vi "RCDAQ Voltage Sweep.vi"() -> ()   [LabVIEW 2023]
doc: "This example shows how to configure a measurement and take a reading."
uses:
  <vilib>/net/SSH/Client/PuTTY/PuTTY Client.lvclass
  C:/Program Files/National Instruments/LabVIEW 2023/vi.lib/net/SSH/Client/Generic/Generic Client.lvclass
  Keithley 2450.lvlib
  <vilib>/net/SSH/NI_SSH.lvlib
panel:
  in  "DRS4 Tme (s)":dbl
  in  "Sweep Points":T1={"Start "=1.0, "Stop "=0.0, "Number of Points (5)"=5}
  out "Error":string
  out "Linux Output":string
  in  "Linux Command":string
  out "Current Voltage":string
  in  "Compliance Level (0.1)":dbl=0.1
  in  "Source Mode  (0: Voltage)":u16(ring) items=["Voltage", "Current"]
  in  "VISA resource name":refnum<visa-resource-name>
  # "(c) 2006 National Instruments.  ALL RIGHTS RESERVED."
  # "(c) 2021 National Instruments.  ALL RIGHTS RESERVED."
  # "Source Settings"
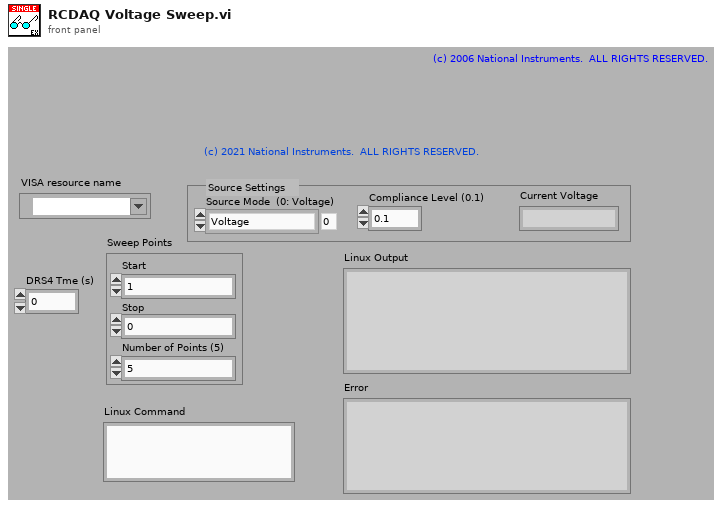
[diagram p1: front panel]
types:
  T1 = cluster{"Start ":dbl, "Stop ":dbl, "Number of Points (5)":u32}
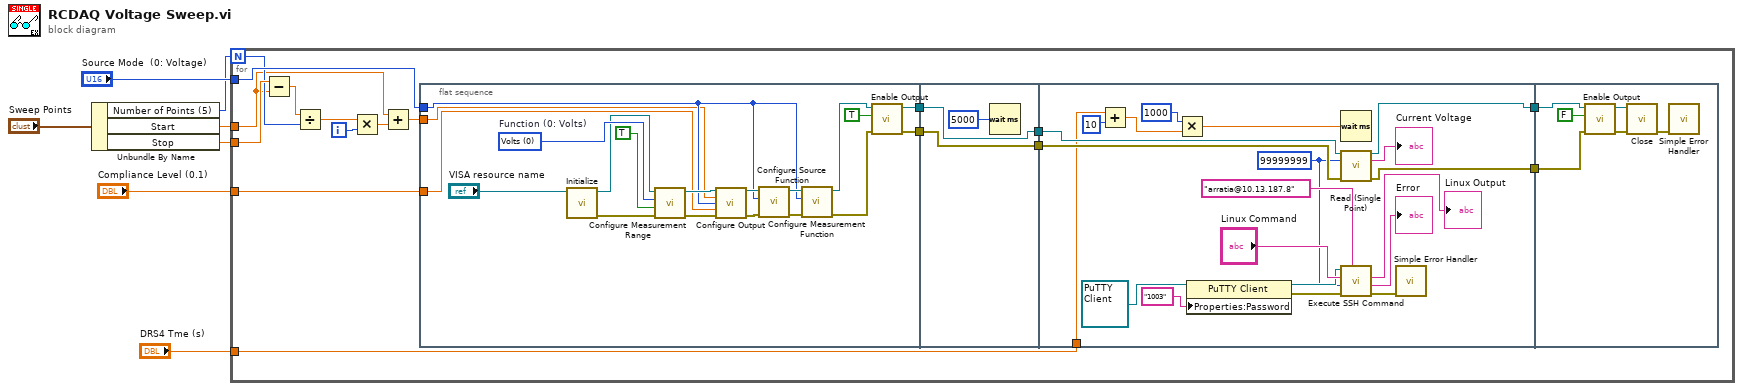
[diagram p0: block diagram]
diagram:
  n1 = Unbundle By Name("Sweep Points") -> ("Number of Points (5)"=w4:u32, "Start"=w3:dbl, "Stop"=w1:dbl)
  n2 = for {
    N: w4 -> [w12]
    tunnel: "Compliance Level (0.1)" -> [w24]
    tunnel: "Source Mode  (0: Voltage)" -> [w23]
    tunnel: w3 -> [w11]
    tunnel: "DRS4 Tme (s)" -> [w15]
    tunnel: w1 -> [w14]
    i -> [w10]
    n3 = Subtract(x=w14, y=w11) -> (x-y=w13:dbl)
    n4 = Divide(x=w13, y=w12) -> (x/y=w9:dbl)
    n5 = Multiply(x=w9, y=w10) -> (x*y=w8:dbl)
    n6 = Add(x=w11, y=w8) -> (x+y=w16:dbl)
    n7 = flat-sequence {
      tunnel: w24 -> [w32]
      tunnel: w23 -> [w31]
      tunnel: [w27] -> w22
      tunnel: [w26] -> w20
      tunnel: w16 -> [w25]
      tunnel: w22 -> [w46]
      tunnel: [w46] -> w21
      tunnel: w20 -> [w45]
      tunnel: [w45] -> w19
      tunnel: w21 -> [w64]
      tunnel: w19 -> [w65]
      tunnel: [w63] -> w18
      tunnel: [w62] -> w17
      tunnel: w15 -> [w50]
      tunnel: w18 -> [w67]
      tunnel: w17 -> [w69]
      frame #0 {
        w40 = u16 0 items=["Volts", "Current", "Resistance"]  # Function (0: Volts)
        n8 = call "Initialize.vi"("VISA resource name"="VISA resource name") -> ("error out"=w38:errorcluster, "VISA resource name out"=w39:refnum<visa-resource-name>)  [unwired: 9 in]
        n9 = call "Configure Measurement Range.vi"("error in (no error)"=w38, "Enable Auto Range (T:Enable)"=TRUE ("Enable Output (T: Enable)"), "Function (0: Volts)"=w40, "VISA resource name"=w39) -> ("error out"=w41:errorcluster, "VISA resource name out"=w42:refnum<visa-resource-name>)  [unwired: 6 in]
        n10 = call "Configure Output.vi"("VISA resource name"=w42, "Source Level (0)"=w25, "Source Mode  (0: Voltage)"=w31, "Source Limit Level (0.1)"=w32, "error in (no error)"=w41) -> ("VISA resource name out"=w37:refnum<visa-resource-name>, "error out"=w36:errorcluster)  [unwired: 9 in]
        n11 = call "Configure Source Function.vi"("error in (no error)"=w36, "Function (0: Volts)"=w31, "VISA resource name"=w37) -> ("error out"=w35:errorcluster, "VISA resource name out"=w34:refnum<visa-resource-name>)  [unwired: 7 in]
        n12 = call "Configure Measurement Function.vi"("error in (no error)"=w35, "Function (0: Volts)"=w31, "VISA resource name"=w34) -> ("error out"=w28:errorcluster, "VISA resource name out"=w29:refnum<visa-resource-name>)  [unwired: 7 in]
        n13 = call "Enable Output.vi"("error in (no error)"=w28, "Enable Output (T: Enable)"=TRUE, "VISA resource name"=w29) -> ("error out"=w27:errorcluster, "VISA resource name out"=w26:refnum<visa-resource-name>)  [unwired: 7 in]
      }
      frame #1 {
        n14 = Wait (ms)(milliseconds to wait=5000) -> ()  [unwired: 1 out]
      }
      frame #2 {
        w47 = 99999999
        n15 = Add(x=w50, y=10) -> (x+y=w49:dbl)
        n16 = Multiply(x=1000, y=w49) -> (x*y=w51:dbl)
        n17 = property class="PuTTY Client"(reference=refnum<class "PuTTY Client.lvclass"> refnum ("NI_SSH.lvlib:PuTTY Client"), "Properties:Password"="1003") -> (reference out=w59:refnum<class "PuTTY Client.lvclass">, error out=w58:errorcluster)  [unwired: 1 in]
        n18 = Wait (ms)(milliseconds to wait=w51) -> ()  [unwired: 1 out]
        n19 = call "Read (Single Point).vi"("VISA resource name"=w65, "Timeout (10000 ms)"=w47, "error in (no error)"=w64) -> ("VISA resource name out"=w63:refnum<visa-resource-name>, "Data out"=→"Current Voltage":string, "error out"=w62:errorcluster)  [unwired: 10 in]
        n20 = call <vilib>:"Execute SSH Command.vi"("user@host"="arratia@10.13.187.8", "error in (no error)"=w58, "timeout (ms)"=w47, "command line"="Linux Command", "session in"=w59) -> ("error out"=w61:errorcluster, "standard error"=→"Error":string, "standard output"=→"Linux Output":string)  [unwired: 2 in, 2 out]
        n21 = call <vilib>:"Simple Error Handler.vi"("error in (no error)"=w61) -> ()  [unwired: 4 in, 5 out]
      }
      frame #3 {
        n22 = call "Enable Output.vi"("error in (no error)"=w69, "Enable Output (T: Enable)"=FALSE, "VISA resource name"=w67) -> ("error out"=w72:errorcluster, "VISA resource name out"=w71:refnum<visa-resource-name>)  [unwired: 7 in]
        n23 = call "Close.vi"("error in (no error)"=w72, "VISA resource name"=w71) -> ("error out"=w70:errorcluster)  [unwired: 9 in]
        n24 = call <vilib>:"Simple Error Handler.vi"("error in (no error)"=w70) -> ()  [unwired: 4 in, 5 out]
      }
    }
  }
